vi "sv_Octave Band Frequencies List.vi"(6 "include units (T)":bool=TRUE, 8 "high band selector":i32, 9 "low band selector":i32, 10 "bandwidth":T3(ring)=enum."1/3 octave", 11 "standard":T1) -> (0 "number of bands":i32, 1 "bandedge frequencies [Hz]":T2(array[cluster]) {"midband" format="%.2f"; "f high" format="%.2f"; "f low" format="%.2f"}, 2 "nominal frequencies (string)":string[](array[string]), 3 "nominal frequencies [Hz]":dbl[](array[numeric]) format="%.2f")   [LabVIEW 2017, in "SoundVib_Octave_2014 standard.lvlib"]
doc: "Returns nominal, or preferred, frequencies and bandedge frequencies based on the specified standard (ANSI or IEC), bandwidth, and low and high band selectors.\nThe frequency range is based on the low and high band selectors. A value of 0 corresponds to the reference frequency of the audio-frequency range, 1 kHz. Each successive value corresponds to the next fractional-octave band. Positive values cover the range above 1 kHz, and negative values cover the range below 1 kHz."
uses:
  <vilib>/addons/Sound and Vibration/svt_Octave/SoundVib_Octave_2014 standard.lvlib
  <vilib>/addons/_NISVFA/_Shared subVIs/Controls/svc_Octave Standard.ctl
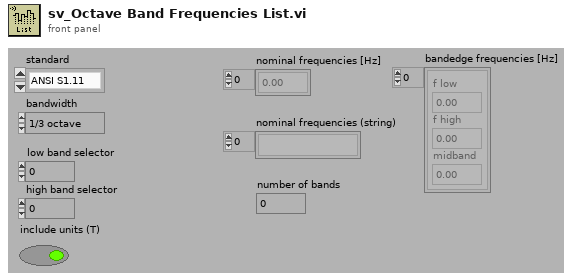
[diagram p1: front panel]
types:
  T1 = typedef "svc_Octave Standard.ctl" = enum16{"ANSI S1.11", "IEC 61260"}
  T2 = cluster{"f low":dbl, "f high":dbl, "midband":dbl}[]
  T3 = enum16{"1 octave", "1/3 octave", "1/6 octave", "1/12 octave", "1/24 octave", "1/48 octave", "1/96 octave"}
  T4 = cluster{"f low":dbl, "f high":dbl, "midband frequency [Hz]":dbl}
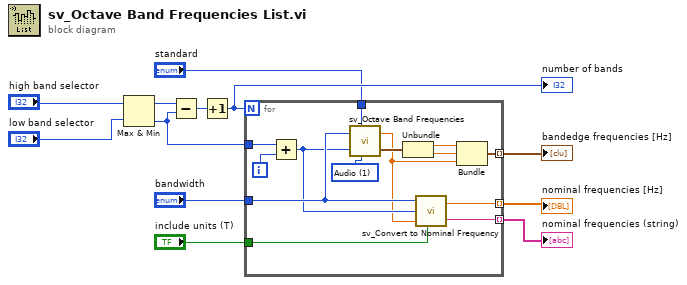
[diagram p0: block diagram]
diagram:
  n1 = Max & Min(x="high band selector", y="low band selector") -> (max(x,y)=w5:i32, min(x,y)=w4:i32)
  n2 = Subtract(x=w5, y=w4) -> (x-y=w12:i32)
  n3 = Increment(x=w12) -> (x+1=w11:i32)
  "number of bands" <- w11
  n4 = for {
    N: w11 -> [_]
    tunnel: w4 -> [w26]
    tunnel: "bandwidth" -> [w18]
    tunnel: [w20] -> w9 mode=indexing
    tunnel: "standard" -> [w19]
    tunnel: [w15] -> w7 mode=indexing
    tunnel: [w14] -> w6 mode=indexing
    tunnel: "include units (T)" -> [w13]
    i -> [w25]
    w24 = u16 1 items=["Infrasonic", "Audio", "Ultrasonic"] ("Frequency range")
    n5 = Add(x=w26, y=w25) -> (x+y=w17:i32)
    n6 = call <vilib>:"sv_Octave Band Frequencies.vi"("octave band selector"=w17, "reference frequency range"=w24, "bandwidth"=w18, "standard"=w19) -> ("bandedge frequencies [Hz]"=w23:cluster{"f low":dbl, "f high":dbl}, "midband frequency [Hz]"=w16:dbl)  [unwired: 2 out]
    n7 = Unbundle(w23) -> ("f low"=w22:dbl, "f high"=w21:dbl)
    n8 = call <vilib>:"sv_Convert to Nominal Frequency.vi"("bandwidth"=w18, "octave band selector"=w17, "midband frequency [Hz]"=w16, "include units (T)"=w13) -> ("nominal frequency [Hz]"=w15:dbl, "nominal frequency (string)"=w14:string)  [unwired: 1 in]
    n9 = Bundle("f low"=w22, "f high"=w21, "midband frequency [Hz]"=w16) -> (w20:T4)  [unwired: 1 in]
  }
  "nominal frequencies [Hz]" <- w7
  "bandedge frequencies [Hz]" <- w9
  "nominal frequencies (string)" <- w6
